vi "labSSH_new_FGGA_Files_Transfer.vi"(0 "Flight_num":string, 1 "Get current?":bool, 5 "Date":string, 7 "Flight Folder Path":path) -> (15 "error IO":errorcluster)   [LabVIEW 2014]
uses:
  <vilib>/Labwerx/labSSH/labSSH.lvlib
panel:
  out "Array of Directory Entries":T1(array[cluster]) {"File Info"."Permissions" format="%o"}
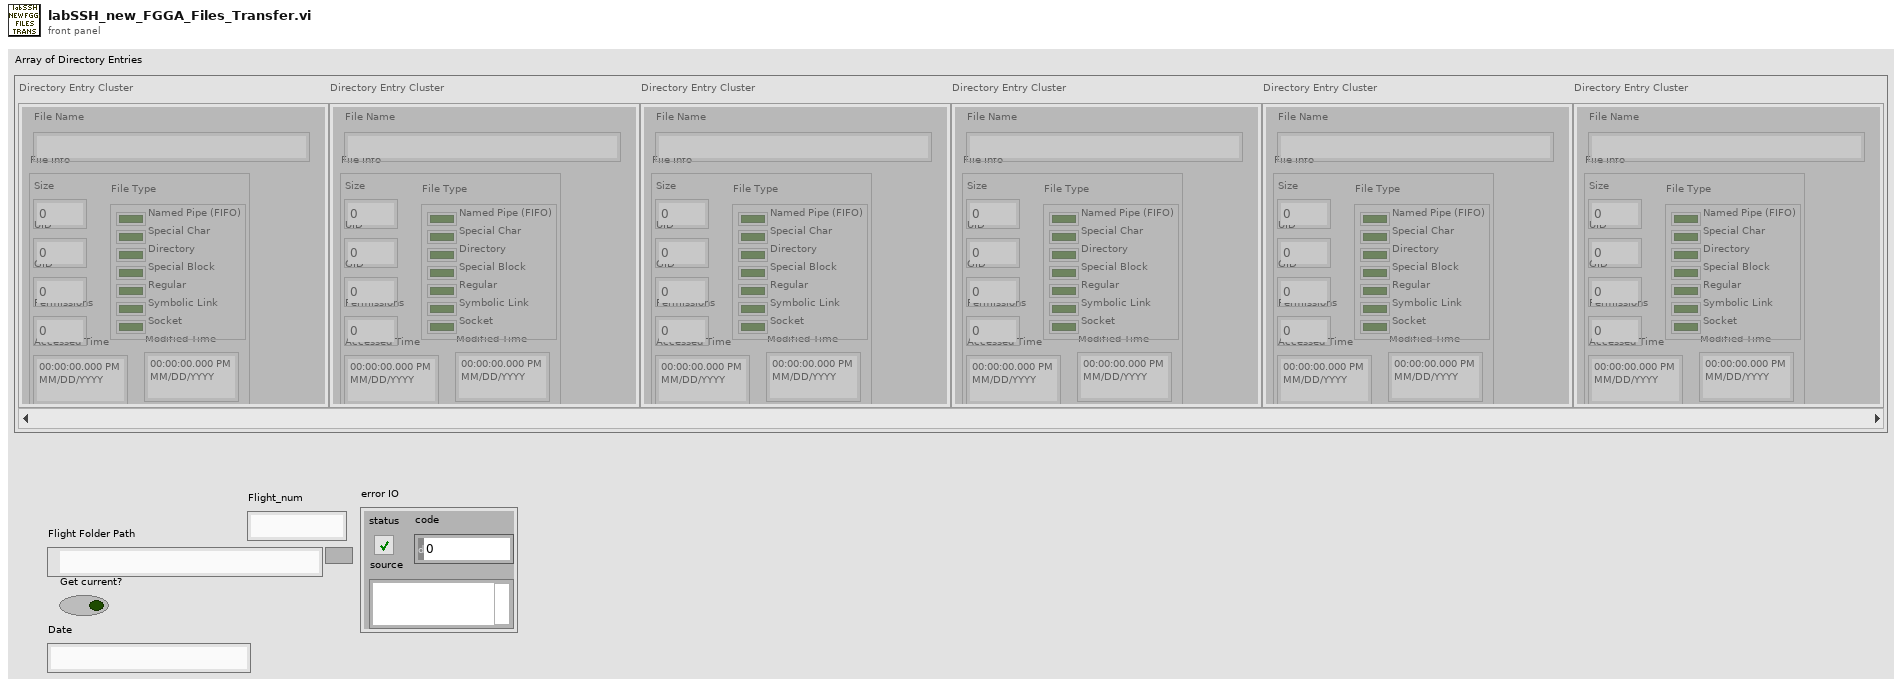
[diagram p1: front panel]
types:
  T1 = cluster{"File Info":cluster{"Size":u32, "UID":u32, "GID":u32, "Permissions":u32, "Accessed Time":timestamp, "Modified Time":timestamp, "File Type":cluster{"Socket":bool, "Directory":bool, "Special Char":bool, "Special Block":bool, "Symbolic Link":bool, "Regular":bool, "Named Pipe (FIFO)":bool}}, "File Name":string}[]
  T2 = enum32{"invalid app kind", "Development System", "Run Time System", "Student Edition", "Embedded LabVIEW", "Evaluation", "Custom"}
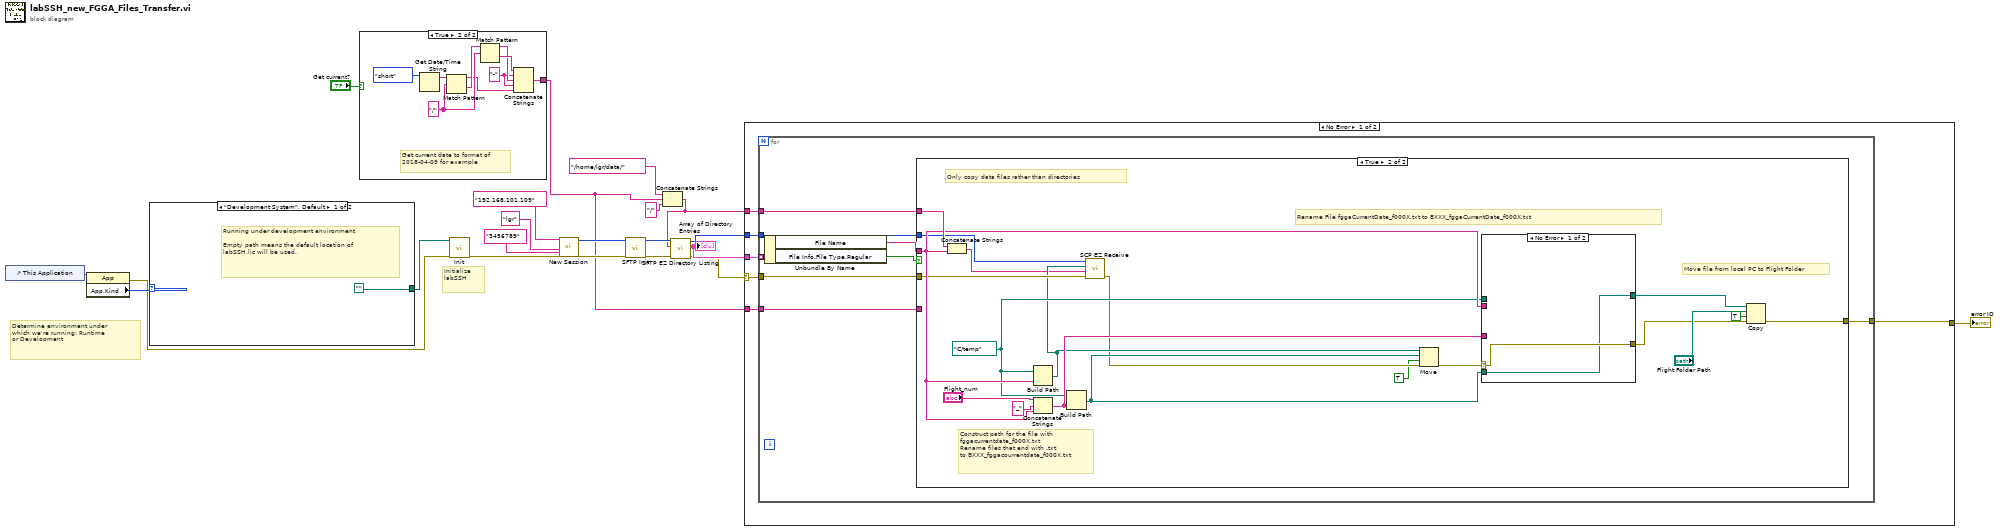
[diagram p0: block diagram]
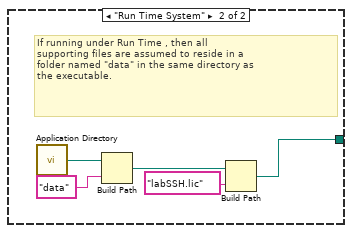
[diagram p2: hidden frame]
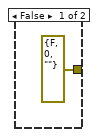
[diagram p3: hidden frame]
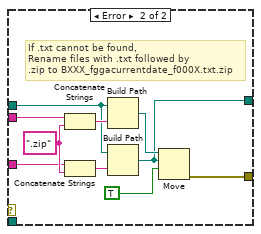
[diagram p4: hidden frame]
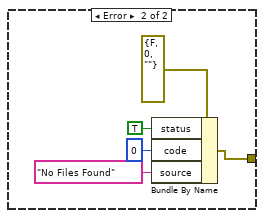
[diagram p5: hidden frame]
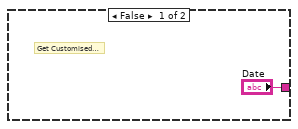
[diagram p6: hidden frame]
diagram:
  # "Initialize \nlabSSH"
  # "Determine environment under\nwhich we're running: Runtime\nor Development"
  n1 = control-ref of="This Application"() -> (w6:refnum<vi>)
  n2 = property class="App"(reference=w6) -> (error out=w3:errorcluster, "App.Kind"=w5:T2)  [unwired: 1 in, 1 out]
  n3 = case shown="\"Development System\", Default" w5 {
    tunnel: [path "" w24] -> w4
    frame "Development System", Default {
      # "Running under development environment\n\nEmpty path means the default location of\nlabSSH.lic will be used."
    }
    frame "Run Time System" {
      # "If running under Run Time , then all\nsupporting files are assumed to reside in a \nfolder named \"data\" in the same directory as\nthe executable."
      n4 = call <vilib>:"Application Directory.vi"() -> ("Application Directory"=w23:path)
      n5 = Build Path(base path=w23, name or relative path="data") -> (appended path=w25:path)
      n6 = Build Path(base path=w25, name or relative path="labSSH.lic") -> (appended path=w24:path)
    }
  }
  n7 = case shown="True" "Get current?" {
    tunnel: ["Date" w29] -> w7
    frame False {
      # "Get Customised Date"
    }
    frame True {
      w31 = "-"
      w34 = "/" ("regular expression")
      # "Get current date to format of\n2018-04-09 for example"
      n8 = Get Date/Time String(date format (0)=enum16{"short", "long", "abbreviated"}."short") -> (date string=w36:string)  [unwired: 2 in, 1 out]
      n9 = Match Pattern(string=w36, regular expression=w34) -> (before substring=w30:string, after substring=w35:string)  [unwired: 1 in, 2 out]
      n10 = Match Pattern(string=w35, regular expression=w34) -> (before substring=w32:string, after substring=w33:string)  [unwired: 1 in, 2 out]
      n11 = Concatenate Strings(w33, w31, w32, w31, w30) -> (w29:string)
    }
  }
  n12 = call <vilib>:"Init.vi"("error in (no error)"=w3, "License File Path Override"=w4) -> ("error out"=w21:errorcluster)  [unwired: 9 in]
  n13 = call <vilib>:"New Session.vi"("IP Addr or Hostname"="192.168.101.109", "Username"="lgr", "Password"="3456789", "error in (no error)"=w21) -> ("New LabSSH Session"=w16:u64, "error out"=w17:errorcluster)  [unwired: 14 in]
  n14 = call <vilib>:"SFTP Init.vi"("error in (no error)"=w17, "LabSSH Session"=w16) -> ("error out"=w14:errorcluster, "LabSSH Session Out"=w15:u64)  [unwired: 8 in]
  n15 = Concatenate Strings("/home/lgr/data/" ("string"), w7, "/" ("string")) -> (w10:string)
  n16 = call <vilib>:"SFTP EZ Directory Listing.vi"("error in (no error)"=w14, "Remote Directory Path"=w10, "LabSSH Session"=w15) -> ("error out"=w8:errorcluster, "Array of Directory Entries"=w12:T1, "LabSSH Session Out"=w11:u64)  [unwired: 5 in, 1 out]
  "Array of Directory Entries" <- w12
  n17 = case shown="No Error" w8 {
    selector: w8 -> [w40 _]
    tunnel: w12 -> [w43 _]
    tunnel: w11 -> [w42 _]
    tunnel: w10 -> [w41 _]
    tunnel: w7 -> [w39 _]
    tunnel: [w38 w84] -> w1
    frame No Error {
      n18 = for {
        tunnel: w43 -> [w51] mode=indexing
        tunnel: w42 -> [w50]
        tunnel: w40 -> [w49]
        tunnel: w41 -> [w48]
        tunnel: w39 -> [w46]
        tunnel: [w44] -> w38
        n19 = Unbundle By Name(w51) -> ("File Name"=w47:string, "File Info.File Type.Regular"=w45:bool)
        n20 = case shown="True" w45 {
          tunnel: w50 -> [_ w63]
          tunnel: w49 -> [_ w64]
          tunnel: w48 -> [_ w71]
          tunnel: w47 -> [_ w67]
          tunnel: w46 -> [_ _]
          tunnel: [errorcluster {"status"=FALSE, "code"=0, "source"=""} ("error out") w53] -> w44
          frame False {
          }
          frame True {
            w66 = path "C:/temp" ("working directory")
            # "Move file from local PC to Flight Folder"
            # "Rename File fggaCurrentDate_f000X.txt to BXXX_fggaCurrentDate_f000X.txt"
            # "Construct path for the file with\nfggacurrentdate_f000X.txt\nRename files that end with .txt\nto BXXX_fggacourrentdate_f000X.txt"
            # "Only copy data files rather than directories"
            n21 = Concatenate Strings(w71, w67) -> (w61:string)
            n22 = Build Path(base path=w66, name or relative path=w67) -> (appended path=w62:path)
            n23 = Concatenate Strings("Flight_num", "_" ("string"), w67) -> (w69:string)
            n24 = Build Path(base path=w66, name or relative path=w69) -> (appended path=w65:path)
            n25 = call <vilib>:"SCP EZ Receive.vi"("error in (no error)"=w64, "Remote Path"=w61, "Local Path"=w62, "LabSSH Session"=w63) -> ("error out"=w60:errorcluster)  [unwired: 3 in, 3 out]
            n26 = Move(source path=w62, error in=w60, 9:TRUE ("overwrite (F)"), 10:w65) -> (error out=w56:errorcluster)  [unwired: 1 in, 2 out]
            n27 = case shown="No Error" w56 {
              selector: w56 -> [w73 _]
              tunnel: w67 -> [_ w83]
              tunnel: w69 -> [_ w79]
              tunnel: [w73 w77] -> w58
              tunnel: [w72 w76] -> w57
              tunnel: w65 -> [w72 _]
              tunnel: w66 -> [_ w74]
              frame No Error {
              }
              frame Error {
                w80 = ".zip" ("string")
                # "If .txt cannot be found,\nRename files with .txt followed by\n.zip to BXXX_fggacurrentdate_f000X.txt.zip"
                n28 = Concatenate Strings(w83, w80) -> (w82:string)
                n29 = Concatenate Strings(w79, w80) -> (w78:string)
                n30 = Build Path(base path=w74, name or relative path=w82) -> (appended path=w81:path)
                n31 = Build Path(base path=w74, name or relative path=w78) -> (appended path=w76:path)
                n32 = Move(source path=w81, 9:TRUE ("overwrite (F)"), 10:w76) -> (error out=w77:errorcluster)  [unwired: 2 in, 2 out]
              }
            }
            n33 = Copy(8:w58, 9:TRUE ("overwrite (F)"), 10:"Flight Folder Path", 11:w57) -> (0:w53:errorcluster)  [unwired: 1 in, 2 out]
          }
        }
      }
    }
    frame Error {
      n34 = Bundle By Name(cluster=errorcluster {"status"=FALSE, "code"=0, "source"=""} ("error IO"), "status"=TRUE, "code"=0, "source"="No Files Found") -> (w84:errorcluster)
    }
  }
  "error IO" <- w1
